vi "remove last plot.vi"   [LabVIEW 2023]
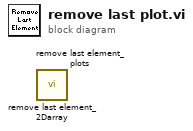
[diagram p0: block diagram]
diagram:
  n1 = call "remove last element_2Darray.vi"() -> ()  [unwired: 11 in, 1 out]
  n2 = call "remove last element_plots.vi"() -> ()  [unwired: 11 in, 1 out]
